vi "Radians to Degrees (Array DBL).vi"(3 "angles (rad)":dbl[](array[numeric]) caption="角（弧度）") -> (1 "angles (deg)":dbl[](array[numeric]) caption="角（角度）")   [LabVIEW 2011, in "NI_AngleManipulation.lvlib"]
doc: "Converts a 1D array of angles from radians to degrees."
uses:
  <vilib>/Utility/AngleManip/NI_AngleManipulation.lvlib
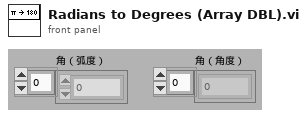
[diagram p1: front panel]
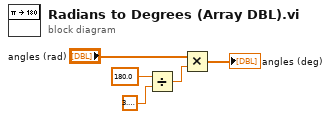
[diagram p0: block diagram]
diagram:
  n1 = Divide(x=180.0 ("y"), y=3.141592653589793) -> (x/y=w3:dbl)
  n2 = Multiply(x="angles (rad)", y=w3) -> (x*y=→"angles (deg)":dbl[])
